vi "cut xy graph using x values.vi"(3 "x_max":sgl, 4 "x_min":sgl, 5 "f(x)":dbl[](array[numeric]), 6 "x":dbl[](array[numeric])) -> (0 "y_cut":dbl[](array[numeric]), 1 "x_cut":dbl[](array[numeric]), 2 "index of start of cut":i32)   [LabVIEW 2013]
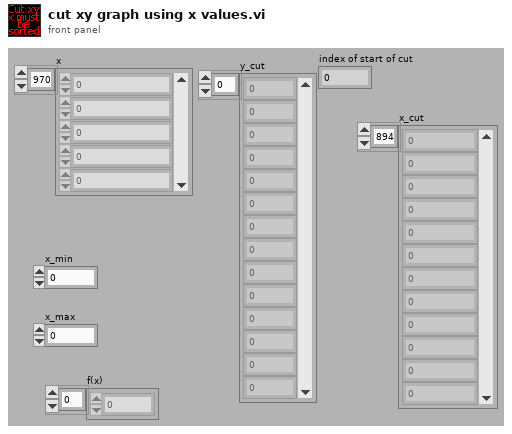
[diagram p1: front panel]
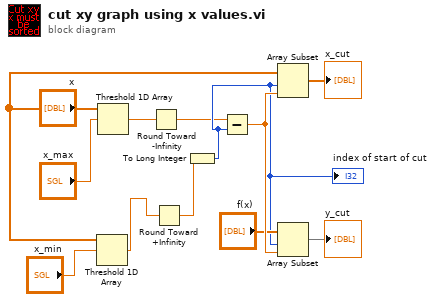
[diagram p0: block diagram]
diagram:
  n1 = Threshold 1D Array(2:"x_min", 3:"x") -> (0:w3:dbl)  [unwired: 1 out]
  n2 = Threshold 1D Array(2:"x_max", 3:"x") -> (0:w8:dbl)  [unwired: 1 out]
  n3 = Round Toward -Infinity(1:w8) -> (0:w1:dbl)
  n4 = Round Toward +Infinity(x=w3) -> (ceil(x): smallest int >= x=w2:dbl)
  n5 = To Long Integer(number=w2) -> (32bit integer=w4:i32)
  "index of start of cut" <- w4
  n6 = Subtract(x=w1, y=w4) -> (x-y=w9:dbl)
  n7 = Array Subset(array="x", index=w4, length=w9) -> (→"x_cut":dbl[])
  n8 = Array Subset(array="f(x)", index=w4, length=w9) -> (→"y_cut":dbl[])
